vi "Undo.vi"(0 "reference in":refnum<class "Client.lvclass">, 5 "Command":T1(ring), 11 "Error In":errorcluster) -> (4 "reference out":refnum<class "Client.lvclass">, 15 "Error Out":errorcluster)   [LabVIEW 2024, in "Client.lvclass"]
doc: "Runs Undo method from IPlayerCommand interface for given command name"
uses:
  Client.lvclass
  Commands/IPlayerCommand_interface/IPlayerCommand.lvclass
panel:
  # "Connector Pane"
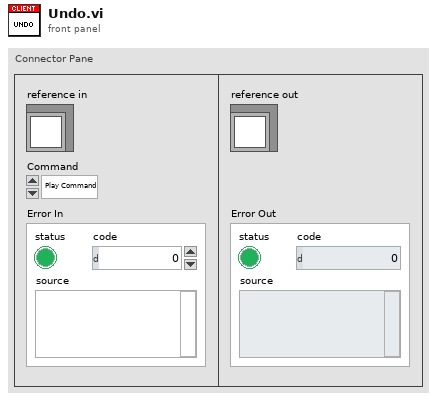
[diagram p1: front panel]
types:
  T1 = enum16{"Play Command", "Pause Command", "Stop Command", "Rewind Command", "Skip Command", ""}
  T2 = typedef "Client.lvclass/ObjectAttributes.ctl" = cluster{"RemoteControlRef":refnum<class "RemoteControl.lvclass">, "MediaPlayerRef":refnum<class "MediaPlayer.lvclass">, "Commands":cluster{"Play Music Command":refnum<class "IPlayerCommand.lvclass">, "Pause Music Command":refnum<class "IPlayerCommand.lvclass">, "Stop Music Command":refnum<class "IPlayerCommand.lvclass">, "Skip Music Command":refnum<class "IPlayerCommand.lvclass">, "Get Current Info Command":refnum<class "IPlayerCommand.lvclass">, "Rewind Music Command":refnum<class "IPlayerCommand.lvclass">}}
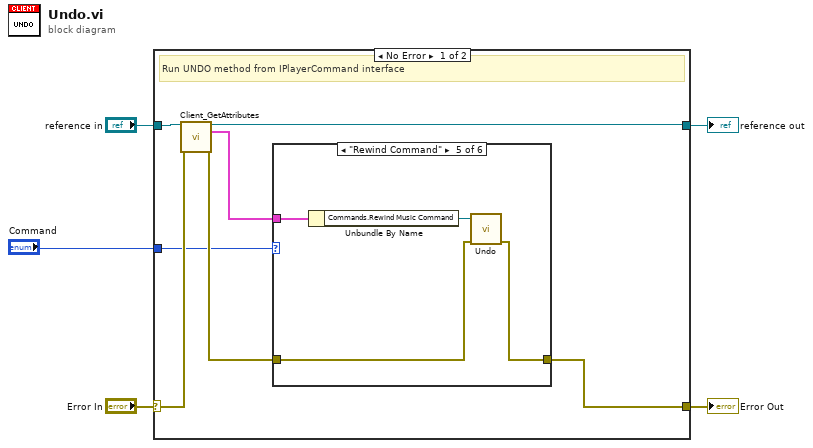
[diagram p0: block diagram]
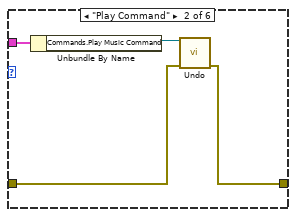
[diagram p3: hidden frame]
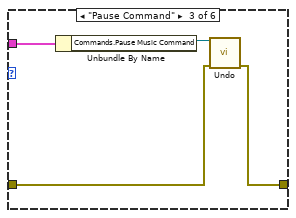
[diagram p4: hidden frame]
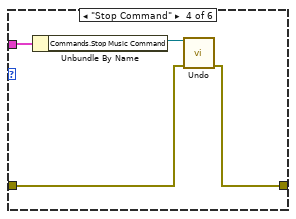
[diagram p5: hidden frame]
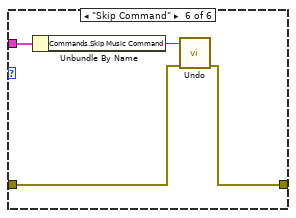
[diagram p6: hidden frame]
diagram:
  n1 = case shown="No Error" "Error In" {
    selector: "Error In" -> [w12 w35]
    tunnel: [w7 w35] -> w4
    tunnel: [w10 w34] -> w2
    tunnel: "reference in" -> [w11 w34]
    tunnel: "Command" -> [w6 _]
    frame No Error {
      # "Run UNDO method from IPlayerCommand interface"
      n2 = call "Client_GetAttributes.vi"("reference in"=w11, "Error In"=w12) -> ("reference out"=w10:refnum<class "Client.lvclass">, "Data"=w9:T2, "Error Out"=w8:errorcluster)  [unwired: 10 in, 1 out]
      n3 = case shown="\"Rewind Command\"" w6 {
        tunnel: w9 -> [_ w16 w21 w22 w29 w33]
        tunnel: w8 -> [w13 w15 w19 w24 w27 w31]
        tunnel: [w13 w14 w18 w23 w26 w32] -> w7
        frame "", Default {
        }
        frame "Play Command" {
          n4 = Unbundle By Name(w16) -> ("Commands.Play Music Command"=w17:refnum<class "IPlayerCommand.lvclass">)
          n5 = call-dynamic "Undo.vi"("object in"=w17, "Error In"=w15) -> ("Error Out"=w14:errorcluster)  [unwired: 12 in, 1 out]
        }
        frame "Pause Command" {
          n6 = Unbundle By Name(w21) -> ("Commands.Pause Music Command"=w20:refnum<class "IPlayerCommand.lvclass">)
          n7 = call-dynamic "Undo.vi"("object in"=w20, "Error In"=w19) -> ("Error Out"=w18:errorcluster)  [unwired: 12 in, 1 out]
        }
        frame "Stop Command" {
          n8 = Unbundle By Name(w22) -> ("Commands.Stop Music Command"=w25:refnum<class "IPlayerCommand.lvclass">)
          n9 = call-dynamic "Undo.vi"("object in"=w25, "Error In"=w24) -> ("Error Out"=w23:errorcluster)  [unwired: 12 in, 1 out]
        }
        frame "Rewind Command" {
          n10 = Unbundle By Name(w29) -> ("Commands.Rewind Music Command"=w28:refnum<class "IPlayerCommand.lvclass">)
          n11 = call-dynamic "Undo.vi"("object in"=w28, "Error In"=w27) -> ("Error Out"=w26:errorcluster)  [unwired: 12 in, 1 out]
        }
        frame "Skip Command" {
          n12 = Unbundle By Name(w33) -> ("Commands.Skip Music Command"=w30:refnum<class "IPlayerCommand.lvclass">)
          n13 = call-dynamic "Undo.vi"("object in"=w30, "Error In"=w31) -> ("Error Out"=w32:errorcluster)  [unwired: 12 in, 1 out]
        }
      }
    }
    frame Error {
    }
  }
  "Error Out" <- w4
  "reference out" <- w2
